vi "Excit_Process_Wfm_And_Name.vi"(8 "error in (no error)":errorcluster, 10 "Excit Number":i32, 11 "EXCIT Waveform Inputs":T1={"Excit Form"=enum."Swift", "Swift Factor"=0.5, "Chirp Apodisation"=3.5, "Duration"=800.0, "Intensity"=100.0, "Start Frequency"=250.0, "End Frequency"=1000.0, "Intensity 2"=100.0, "Start Frequency 2"=250.0, "End Frequency 2"=350.0, "Sampling Frequency"=10.0} {"End Frequency 2" min=1.0 max=10000.0; "Start Frequency 2" min=1.0 max=10000.0; "Intensity 2" min=1.0 max=100.0; "Chirp Apodisation" min=1.0 max=5.0 step=0.1; "Swift Factor" min=0.1 max=3.0 step=0.1; "Sampling Frequency" min=1.0 max=100.0 step=1.0; "Duration" min=1.0 max=1000000.0 step=1.0; "End Frequency" min=1.0 max=10000.0; "Start Frequency" min=1.0 max=10000.0 step=0.1 format="%#.6g"; "Intensity" min=1.0 max=100.0}) -> (0 "error out":errorcluster caption="sortie d'erreur", 1 "FIFO used":i32, 2 "Excitation FFT":cluster{dbl[], "Power Spectrum (V^2 rms)":dbl[]}(graph), 3 "Excitation Signal":T2(graph), 4 "Waveform Name":string, 5 "Signal Excitation":dbl[](array[numeric]))   [LabVIEW 2017]
uses:
  controls/EXCIT_Waveform_Inputs.ctl
  <vilib>/Analysis/NI_AALPro.lvlib
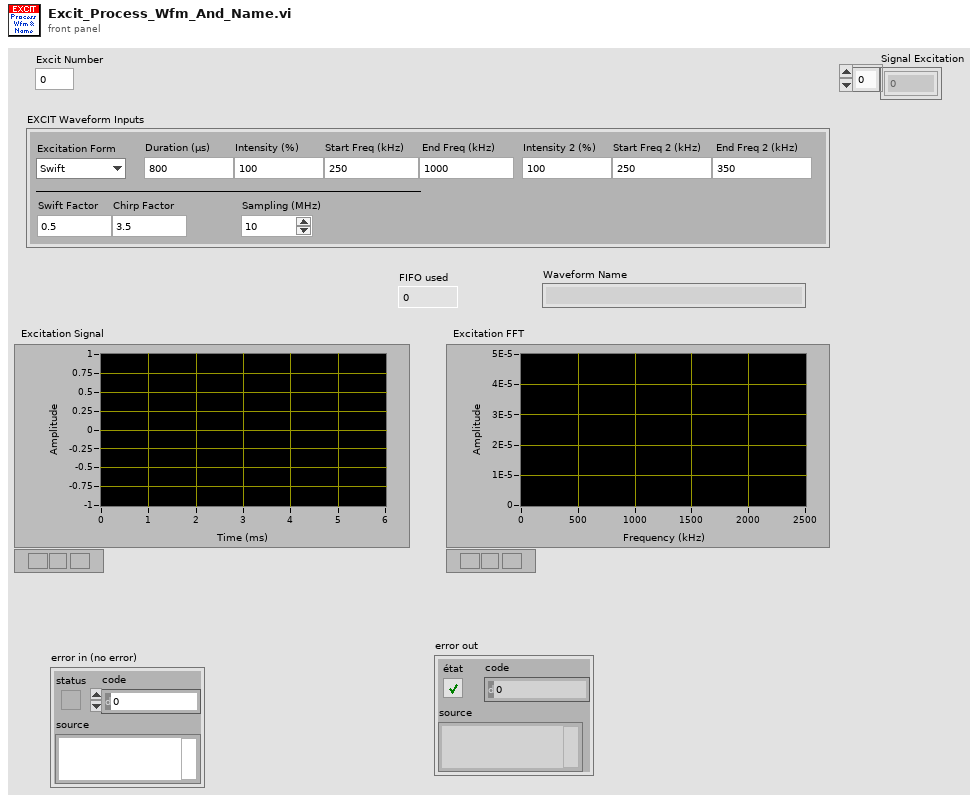
[diagram p1: front panel]
types:
  T1 = typedef "EXCIT_Waveform_Inputs.ctl" = cluster{"Excit Form":enum16{"Sinus", "Chirp", "Swift", "TwoSwift", "Ramp"}, "Swift Factor":dbl, "Chirp Apodisation":dbl, "Duration":dbl, "Intensity":dbl, "Start Frequency":dbl, "End Frequency":dbl, "Intensity 2":dbl, "Start Frequency 2":dbl, "End Frequency 2":dbl, "Sampling Frequency":dbl}
  T2 = cluster{"X Time":dbl[], "Signal Excitation":dbl[]}
  T3 = enum16{"Sinus", "Chirp", "Swift", "TwoSwift", "Ramp"}
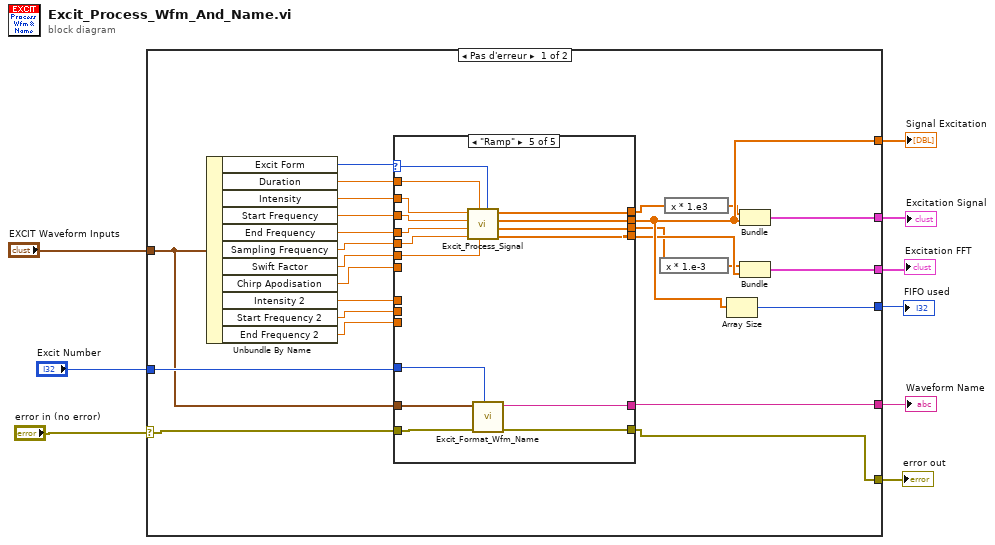
[diagram p0: block diagram]
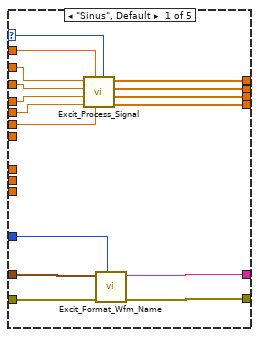
[diagram p2: hidden frame]
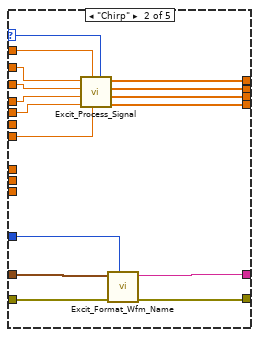
[diagram p3: hidden frame]
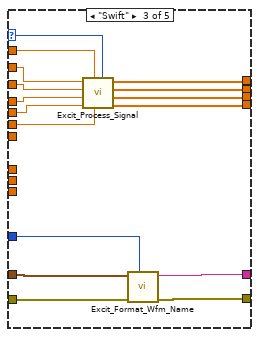
[diagram p4: hidden frame]
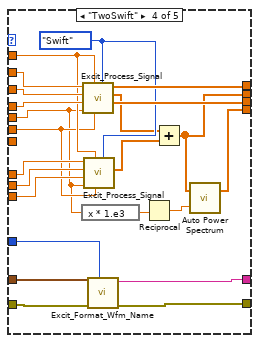
[diagram p5: hidden frame]
diagram:
  n1 = case shown="Pas d'erreur" "error in (no error)" {
    selector: "error in (no error)" -> [w14 _]
    tunnel: [w34 _] -> w9
    tunnel: "Excit Number" -> [w32 _]
    tunnel: [w31 _] -> w7
    tunnel: [w15 _] -> w6
    tunnel: "EXCIT Waveform Inputs" -> [w13 _]
    tunnel: [w12 _] -> w3
    tunnel: [w11 _] -> w2
    tunnel: [w10 _] -> w1
    frame No Error {
      n2 = Unbundle By Name(w13) -> ("Excit Form"=w33:T3, "Duration"=w18:dbl, "Intensity"=w19:dbl, "Start Frequency"=w20:dbl, "End Frequency"=w21:dbl, "Sampling Frequency"=w22:dbl, "Swift Factor"=w23:dbl, "Chirp Apodisation"=w24:dbl, "Intensity 2"=w28:dbl, "Start Frequency 2"=w29:dbl, "End Frequency 2"=w30:dbl)
      n3 = case shown="\"Ramp\"" w33 {
        selector: w33 -> [w50 w66 w82 _ w117]
        tunnel: w24 -> [_ w51 _ _ _]
        tunnel: w18 -> [w40 w56 w73 w89 w111]
        tunnel: w19 -> [w39 w55 w72 w92 w110]
        tunnel: w20 -> [w38 w54 w71 w91 w109]
        tunnel: w21 -> [w37 w53 w70 w90 w108]
        tunnel: w22 -> [w36 w52 w69 w84 w107]
        tunnel: w23 -> [w35 _ w68 w85 w106]
        tunnel: [w49 w65 w81 w105 w121] -> w25
        tunnel: [w48 w64 w80 w99 w120] -> w31
        tunnel: [w47 w63 w79 w104 w119] -> w26
        tunnel: [w46 w62 w78 w97 w118] -> w27
        tunnel: w28 -> [_ _ _ w88 _]
        tunnel: w29 -> [_ _ _ w87 _]
        tunnel: w30 -> [_ _ _ w86 _]
        tunnel: [w43 w58 w75 w93 w115] -> w15
        tunnel: [w42 w59 w74 w94 w113] -> w34
        tunnel: w14 -> [w44 w60 w76 w95 w116]
        tunnel: w32 -> [w45 w61 w77 w96 w114]
        tunnel: w13 -> [w41 w57 w67 w83 w112]
        frame "Sinus", Default {
          n4 = call "Excit_Process_Signal.vi"("Excit Form"=w50, "Factor"=w35, "Duration (µs)"=w40, "Sampling Frequency (MHz)"=w36, "End Frequency (kHz)"=w37, "Start Frequency (kHz)"=w38, "Amplitude (%)"=w39) -> ("FFT Excitation"=w46:dbl[], "X Freq"=w47:dbl[], "Signal Excitation"=w48:dbl[], "X Time"=w49:dbl[])
          n5 = call "Excit_Format_Wfm_Name.vi"("Excit Number"=w45, "error in"=w44, "EXCIT Waveforms Inputs"=w41) -> ("error out"=w43:errorcluster, "Waveform Name"=w42:string)  [unwired: 7 in]
        }
        frame "Chirp" {
          n6 = call "Excit_Process_Signal.vi"("Excit Form"=w66, "Factor"=w51, "Duration (µs)"=w56, "Sampling Frequency (MHz)"=w52, "End Frequency (kHz)"=w53, "Start Frequency (kHz)"=w54, "Amplitude (%)"=w55) -> ("FFT Excitation"=w62:dbl[], "X Freq"=w63:dbl[], "Signal Excitation"=w64:dbl[], "X Time"=w65:dbl[])
          n7 = call "Excit_Format_Wfm_Name.vi"("Excit Number"=w61, "error in"=w60, "EXCIT Waveforms Inputs"=w57) -> ("error out"=w58:errorcluster, "Waveform Name"=w59:string)  [unwired: 7 in]
        }
        frame "Swift" {
          n8 = call "Excit_Process_Signal.vi"("Excit Form"=w82, "Factor"=w68, "Duration (µs)"=w73, "Sampling Frequency (MHz)"=w69, "End Frequency (kHz)"=w70, "Start Frequency (kHz)"=w71, "Amplitude (%)"=w72) -> ("FFT Excitation"=w78:dbl[], "X Freq"=w79:dbl[], "Signal Excitation"=w80:dbl[], "X Time"=w81:dbl[])
          n9 = call "Excit_Format_Wfm_Name.vi"("Excit Number"=w77, "error in"=w76, "EXCIT Waveforms Inputs"=w67) -> ("error out"=w75:errorcluster, "Waveform Name"=w74:string)  [unwired: 7 in]
        }
        frame "TwoSwift" {
          w103 = T3."Swift" ("Excit Form")
          n10 = expression code="x * 1.e3"(w84) -> (w100:dbl)
          n11 = call "Excit_Process_Signal.vi"("Excit Form"=w103, "Factor"=w85, "Duration (µs)"=w89, "Sampling Frequency (MHz)"=w84, "End Frequency (kHz)"=w90, "Start Frequency (kHz)"=w91, "Amplitude (%)"=w92) -> ("X Freq"=w104:dbl[], "Signal Excitation"=w102:dbl[], "X Time"=w105:dbl[])  [unwired: 1 out]
          n12 = call "Excit_Process_Signal.vi"("Excit Form"=w103, "Factor"=w85, "Duration (µs)"=w89, "Sampling Frequency (MHz)"=w84, "End Frequency (kHz)"=w86, "Start Frequency (kHz)"=w87, "Amplitude (%)"=w88) -> ("Signal Excitation"=w101:dbl[])  [unwired: 3 out]
          n13 = call "Excit_Format_Wfm_Name.vi"("Excit Number"=w96, "error in"=w95, "EXCIT Waveforms Inputs"=w83) -> ("error out"=w93:errorcluster, "Waveform Name"=w94:string)  [unwired: 7 in]
          n14 = Reciprocal(x=w100) -> (1/x=w98:dbl)
          n15 = Add(x=w102, y=w101) -> (x+y=w99:dbl[])
          n16 = call <vilib>:"Auto Power Spectrum.vi"("dt"=w98, "Signal (V)"=w99) -> ("Power Spectrum (V^2 rms)"=w97:dbl[])  [unwired: 1 out]
        }
        frame "Ramp" {
          n17 = call "Excit_Process_Signal.vi"("Excit Form"=w117, "Factor"=w106, "Duration (µs)"=w111, "Sampling Frequency (MHz)"=w107, "End Frequency (kHz)"=w108, "Start Frequency (kHz)"=w109, "Amplitude (%)"=w110) -> ("FFT Excitation"=w118:dbl[], "X Freq"=w119:dbl[], "Signal Excitation"=w120:dbl[], "X Time"=w121:dbl[])
          n18 = call "Excit_Format_Wfm_Name.vi"("Excit Number"=w114, "error in"=w116, "EXCIT Waveforms Inputs"=w112) -> ("error out"=w115:errorcluster, "Waveform Name"=w113:string)  [unwired: 7 in]
        }
      }
      n19 = expression code="x * 1.e-3"(w26) -> (w17:dbl[])
      n20 = expression code="x * 1.e3"(w25) -> (w16:dbl[])
      n21 = Array Size(array=w31) -> (size(s)=w10:i32)
      n22 = Bundle("X Time"=w16, "Signal Excitation"=w31) -> (w12:T2)  [unwired: 1 in]
      n23 = Bundle("X Freq"=w17, "FFT Excitation"=w27) -> (w11:cluster{"X Freq":dbl[], "FFT Excitation":dbl[]})  [unwired: 1 in]
    }
    frame Error {
    }
  }
  "Waveform Name" <- w9
  "Signal Excitation" <- w7
  "error out" <- w6
  "Excitation Signal" <- w3
  "Excitation FFT" <- w2
  "FIFO used" <- w1
